vi "Write Device Type.vi"(8 "error in (no error)":errorcluster, 10 "Device Type":T1, 11 "Generic Device in":refnum<class "Generic Device.lvclass">) -> (0 "error out":errorcluster, 3 "Generic Device out":refnum<class "Generic Device.lvclass">)   [LabVIEW 2014, in "Generic Device.lvlib" / "Generic Device.lvclass"]
uses:
  Generic Device.lvclass
  Controls/Generic Device Type.ctl
  Generic Device.lvclass/Generic Device.ctl
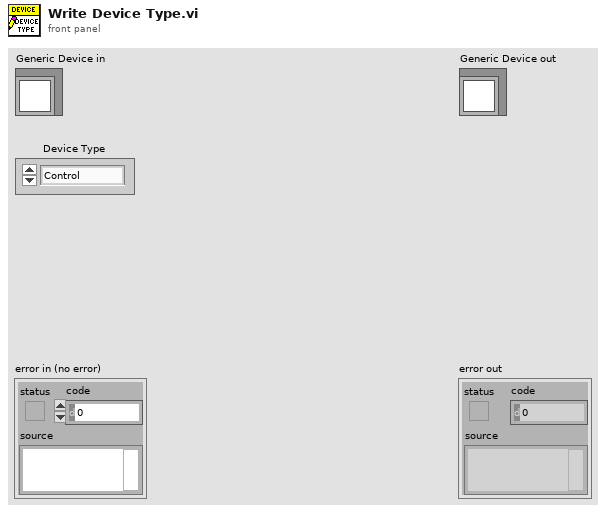
[diagram p1: front panel]
types:
  T1 = typedef "Generic Device Type.ctl" = enum16{"Control", "Instrument"}
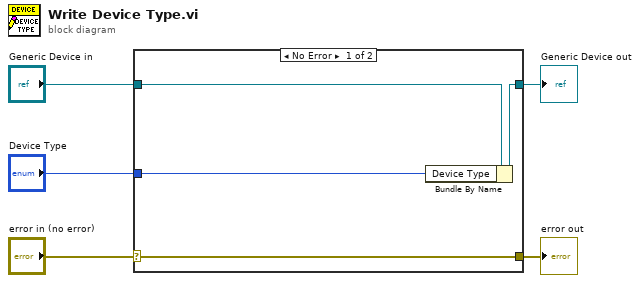
[diagram p0: block diagram]
diagram:
  n1 = case shown="No Error" "error in (no error)" {
    selector: "error in (no error)" -> [w9 w10]
    tunnel: [w9 w10] -> w4
    tunnel: [w7 w11] -> w2
    tunnel: "Generic Device in" -> [w8 w11]
    tunnel: "Device Type" -> [w6 _]
    frame No Error {
      n2 = Bundle By Name(cluster=w8, "Device Type"=w6) -> (w7:refnum<class "Generic Device.lvclass">)
    }
    frame Error {
    }
  }
  "error out" <- w4
  "Generic Device out" <- w2
